vi "add volume by URL.vi"(5 "volume parent dir":path, 7 "issue parent dir":path, 8 "error in (no error)":errorcluster, 10 "URL":string, 11 "ComicVine_manager in":refnum<class "CV_downloader.lvclass">) -> (0 "error out":errorcluster, 3 "ComicVine_manager out":refnum<class "CV_downloader.lvclass">)   [LabVIEW 2024, in "CV_downloader.lvclass"]
uses:
  CV_downloader.lvclass
  WebScraper/series_class/series_class.lvclass
  C:/code/LabVIEW_Projects/applications/ComicVine_API/WebScraper/comic_class/comic_class.lvclass
  WebScraper/series_class/series_class.lvclass/series_class.ctl
  WebScraper/comic_class/comic_class.lvclass
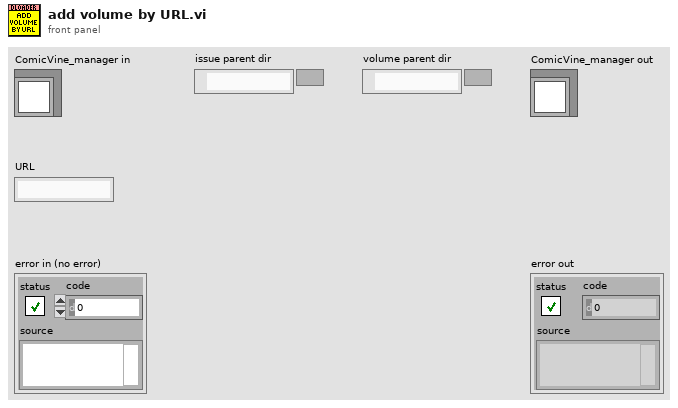
[diagram p1: front panel]
types:
  T1 = typedef "issueInfo.ctl" = cluster{"cover date":timestamp, "release date":timestamp, "number":string, "url":string, "small cover url":string, "name":string, "large cover url":string, "id":string, "creators":T2[], "characters":T3[], "teams":T4[], "locations":T5[], "concepts":T6[], "objects":T7[], "storyArcs":T8[], "description":string}
  T2 = typedef "creator.ctl" = cluster{"name":string, "role":string, "url":string}
  T3 = typedef "character.ctl" = cluster{"name":string, "url":string}
  T4 = typedef "team.ctl" = cluster{"name":string, "url":string}
  T5 = typedef "location.ctl" = cluster{"name":string, "url":string}
  T6 = typedef "concept.ctl" = cluster{"name":string, "url":string}
  T7 = typedef "thing.ctl" = cluster{"name":string, "url":string}
  T8 = typedef "storyArc.ctl" = cluster{"name":string, "url":string}
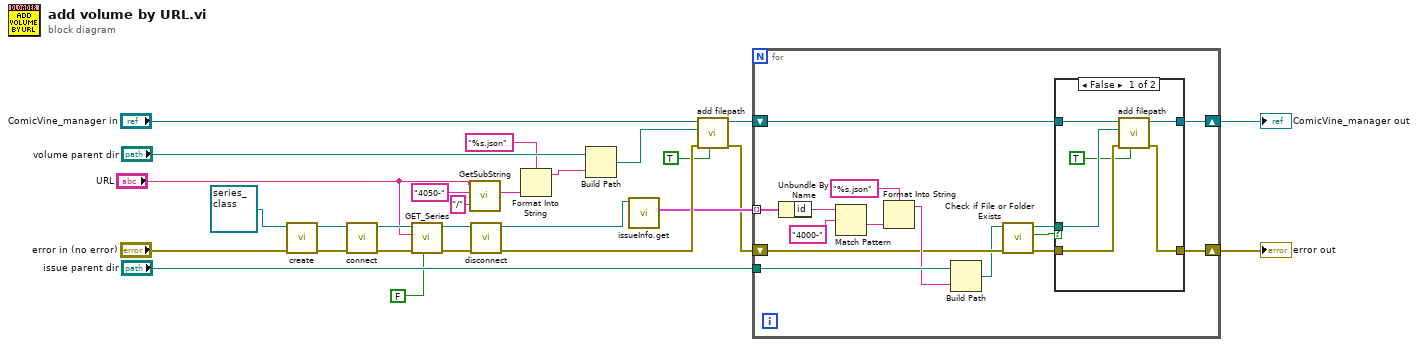
[diagram p0: block diagram]
diagram:
  n1 = call "create.vi"("error in (no error)"="error in (no error)", "comic_class in"=refnum<class "series_class.lvclass"> refnum ("series_class.lvclass")) -> ("error out"=w24:errorcluster, "comic_class out"=w25:refnum<class "series_class.lvclass">)  [unwired: 8 in]
  n2 = call-dynamic "connect.vi"("error in (no error)"=w24, "comic_class in"=w25) -> ("error out"=w22:errorcluster, "comic_class out"=w23:refnum<class "series_class.lvclass">)  [unwired: 8 in]
  n3 = call "GET_Series.vi"("get all issues"=FALSE, "error in (no error)"=w22, "series URL"="URL", "ComicVine_class in"=w23) -> ("error out"=w19:errorcluster, "ComicVine_class out"=w20:refnum<class "series_class.lvclass">)  [unwired: 6 in]
  n4 = call "GetSubString.vi"("End Search"="/", "Start Search"="4050-" ("regular expression"), "String In"="URL") -> ("Match"=w4:string)  [unwired: 6 in, 2 out]
  n5 = call-dynamic "disconnect.vi"("error in (no error)"=w19, "comic_class in"=w20) -> ("error out"=w15:errorcluster, "comic_class out"=w18:refnum<class "series_class.lvclass">)  [unwired: 8 in]
  n6 = Format Into String(format string="%s.json", w4) -> (resulting string=w2:string)  [unwired: 2 in, 1 out]
  n7 = Build Path(base path="volume parent dir", name or relative path=w2) -> (appended path=w16:path)
  n8 = call "issueInfo.get.vi"("ComicVine_class in"=w18) -> ("issueInfo"=w13:T1[])  [unwired: 9 in, 1 out]
  n9 = call "add filepath.vi"("priority (F)"=TRUE, "error in (no error)"=w15, "filepath"=w16, "ComicVine_manager in"="ComicVine_manager in") -> ("error out"=w11:errorcluster, "ComicVine_manager out"=w10:refnum<class "CV_downloader.lvclass">)  [unwired: 6 in]
  n10 = for {
    tunnel: w13 -> [w42] mode=indexing
    tunnel: "issue parent dir" -> [w37]
    shift-right: [w31] -> w8
    shift-left: w11 -> [w35]
    shift-right: [w29] -> w9
    shift-left: w10 -> [w30]
    n11 = Unbundle By Name(w42) -> ("id"=w41:string)
    n12 = Match Pattern(string=w41, regular expression="4000-") -> (after substring=w39:string)  [unwired: 1 in, 3 out]
    n13 = Format Into String(format string="%s.json", w39) -> (resulting string=w36:string)  [unwired: 2 in, 1 out]
    n14 = Build Path(base path=w37, name or relative path=w36) -> (appended path=w34:path)
    n15 = call <vilib>:"Check if File or Folder Exists.vi"("error in (no error)"=w35, "path"=w34) -> ("error out"=w32:errorcluster, "file or folder exists?"=w33:bool, "dup path"=w28:path)  [unwired: 7 in]
    n16 = case shown="False" w33 {
      tunnel: w32 -> [w46 w50]
      tunnel: [w45 w50] -> w31
      tunnel: [w44 w49] -> w29
      tunnel: w30 -> [w48 w49]
      tunnel: w28 -> [w47 _]
      frame False {
        n17 = call "add filepath.vi"("priority (F)"=TRUE, "error in (no error)"=w46, "filepath"=w47, "ComicVine_manager in"=w48) -> ("error out"=w45:errorcluster, "ComicVine_manager out"=w44:refnum<class "CV_downloader.lvclass">)  [unwired: 6 in]
      }
      frame True {
      }
    }
  }
  "error out" <- w8
  "ComicVine_manager out" <- w9
